vi "Untitled 3.vi"() -> ()   [LabVIEW 2022 SP3]
panel:
  out "value 2":string
  out "value":cluster{"wode":string}
  out "JSON string":string
  out "String":string
  out "unsigned byte array":u8[](array[numeric])
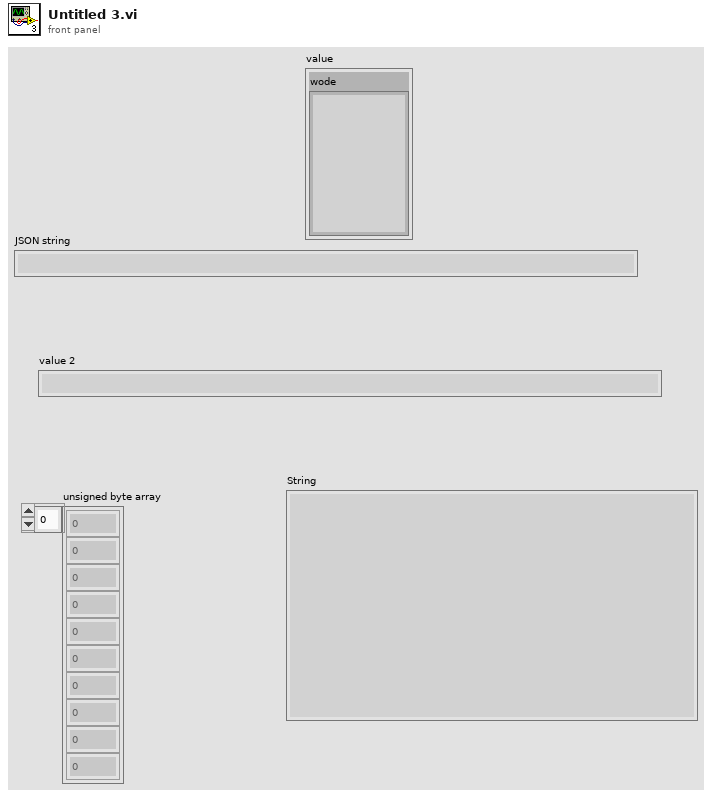
[diagram p1: front panel]
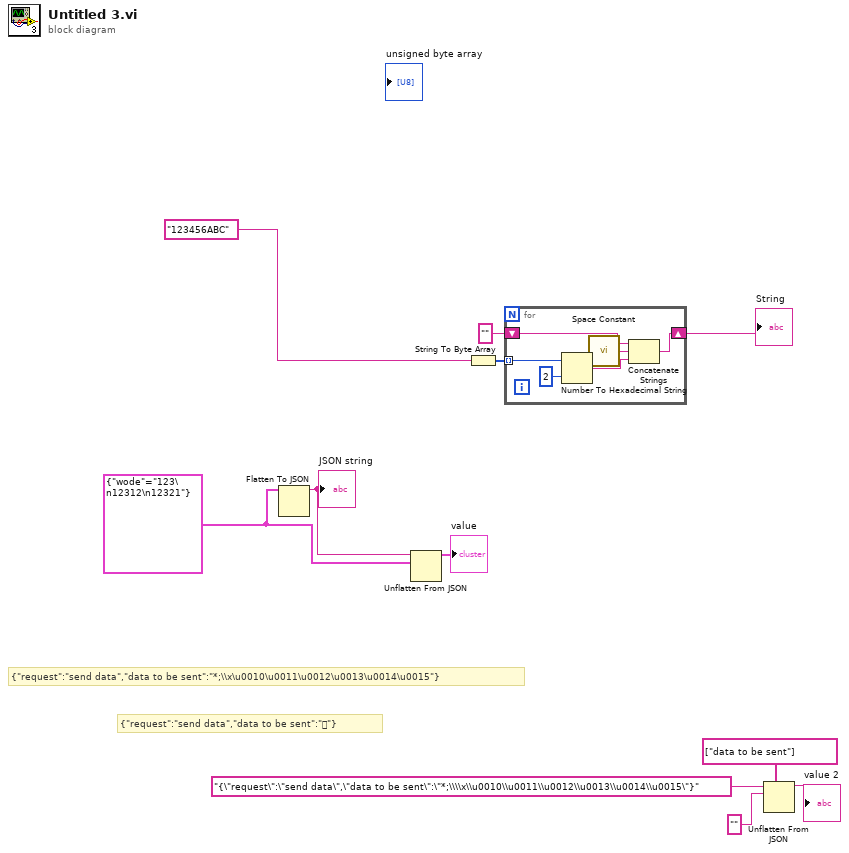
[diagram p0: block diagram]
diagram:
  w6 = cluster{"wode":string} {"wode"="123\n12312\n12321"}
  # "{\"request\":\"send data\",\"data to be sent\":\"\"}"
  # "{\"request\":\"send data\",\"data to be sent\":\"*;\\\\x\\u0010\\u0011\\u0012\\u0013\\u0014\\u0015\"}"
  n1 = Flatten To JSON(anything=w6) -> (JSON string=w7:string)  [unwired: 2 in, 1 out]
  "JSON string" <- w7
  n2 = Unflatten From JSON(JSON string=w7, type and defaults=w6) -> (value=→"value":cluster{"wode":string})  [unwired: 5 in, 1 out]
  n3 = String To Byte Array(string="123456ABC") -> (unsigned byte array=w8:u8[])
  n4 = for {
    tunnel: w8 -> [w16] mode=indexing
    shift-right: [w14] -> w9
    shift-left: "" -> [w15]
    n5 = Number To Hexadecimal String(1:i16 2 ("width (-)"), 2:w16) -> (0:w13:string)
    n6 = call <vilib>:"Space Constant.vi"() -> ("String"=w12:string)
    n7 = Concatenate Strings(w15, w12, w13) -> (w14:string)
  }
  "String" <- w9
  n8 = Unflatten From JSON(path=string[] ["data to be sent"], JSON string="{\"request\":\"send data\",\"data to be sent\":\"*;\\\\x\\u0010\\u0011\\u0012\\u0013\\u0014\\u0015\"}", type and defaults="") -> (value=→"value 2":string)  [unwired: 4 in, 1 out]
